vi "Set Formatter.vi"(8 "error in":errorcluster, 10 "Formatter.lvclass":refnum<class "Formatter.lvclass">, 11 "FileHandler":refnum<class "NetworkHandler.lvclass">) -> (0 "error out":errorcluster, 3 "FileHandler out":refnum<class "NetworkHandler.lvclass">)   [LabVIEW 2024]
doc: "Sets the Formatter for this handler to fmt.\n\n____\nHAMPEL SOFTWARE ENGINEERING v2.2.2 (2025-01-16 15:41)"
uses:
  <vilib>/Hampel Software Engineering/HSE Logger/Formatter/Formatter.lvclass
  NetworkHandler.lvclass
  NetworkHandler.lvclass/NetworkHandler.ctl
  C:/Program Files (x86)/National Instruments/LabVIEW 2024/vi.lib/Hampel Software Engineering/HSE Logger/Handler/Handler.lvclass
  C:/DevOps/CORTEX/X_T2126_SDE_Rig_CAT/HSEExtensions/NetworkHandler/NetworkHandler.lvclass
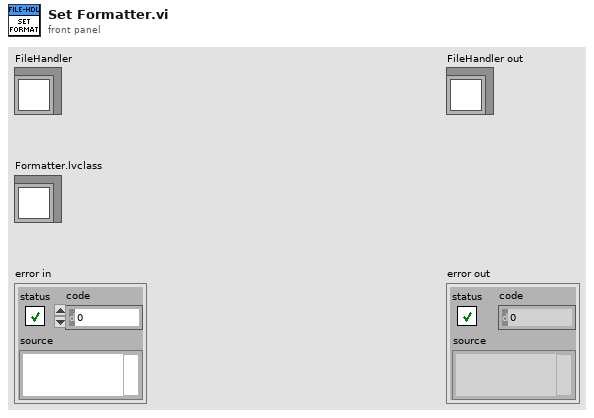
[diagram p1: front panel]
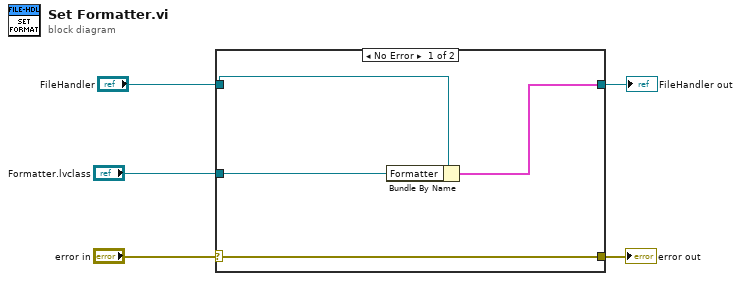
[diagram p0: block diagram]
diagram:
  n1 = case shown="No Error" "error in" {
    selector: "error in" -> [w9 w11]
    tunnel: [w9 w11] -> w4
    tunnel: [w7 w10] -> w1
    tunnel: "FileHandler" -> [w8 w10]
    tunnel: "Formatter.lvclass" -> [w6 _]
    frame No Error {
      n2 = Bundle By Name(cluster=w8, "Formatter"=w6) -> (w7:cluster{})
    }
    frame Error {
    }
  }
  "error out" <- w4
  "FileHandler out" <- w1
